vi "SRV_Comm.vi"(3 "TCP Settings":T1={"Method"=enum."General", "bytes to read"=2000, "timeout ms (1000)"=1000}, 4 "Command Sent":string, 5 "SRV In":refnum<k5>) -> (0 "Full comm":string, 1 "Reply":string, 2 "SRV Out":refnum<k5>)   [LabVIEW 2009]
uses:
  SRVGlobals.vi
  TCP_Communication/SRV_TCP Settings.ctl
  TCP_Communication/SRV_Package Methods.ctl
panel:
  # "This LabVIEW item is deprecated.\n\nIt is believed to be unused and will be removed in a future version of SRV."
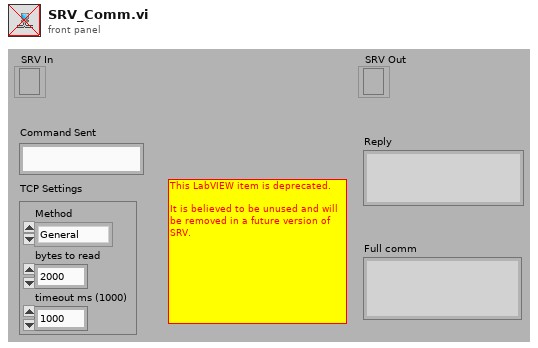
[diagram p1: front panel]
types:
  T1 = typedef "SRV_TCP Settings.ctl" = cluster{"Method":T2, "bytes to read":i32, "timeout ms (1000)":i32}
  T2 = typedef "SRV_Package Methods.ctl" = enum16{"General", "Standard", "CRLF", "Image", "HTML"}
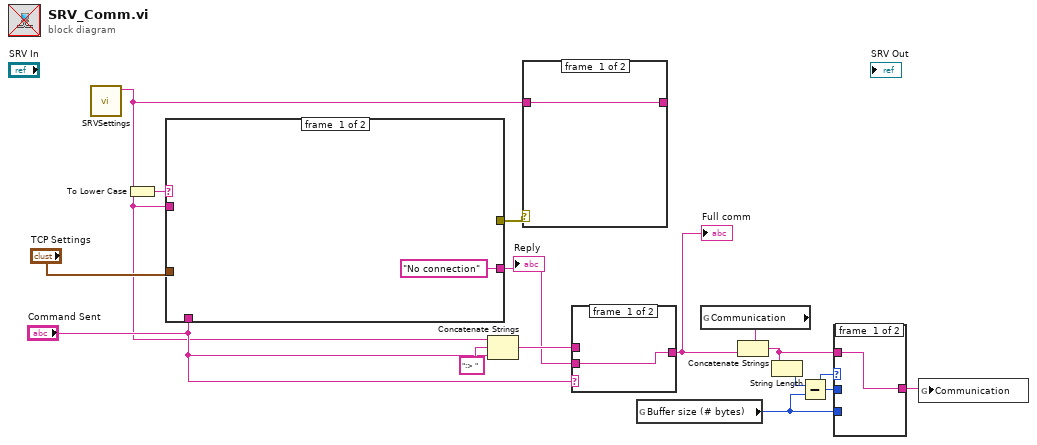
[diagram p0: block diagram]
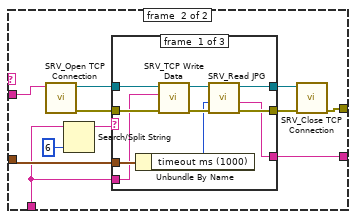
[diagram p2: hidden frame]
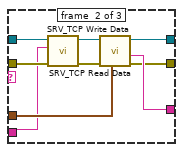
[diagram p3: hidden frame]
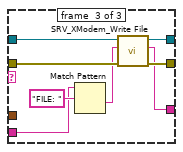
[diagram p4: hidden frame]
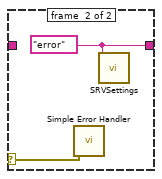
[diagram p5: hidden frame]
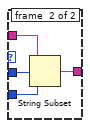
[diagram p6: hidden frame]
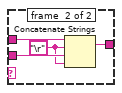
[diagram p7: hidden frame]
diagram:
  n1 = call "SRVSettings.vi"() -> ("SRV IP Address out"=w2:string, "SRV IP Address"=w5:string)  [unwired: 8 in, 2 out]
  n2 = To Lower Case(string=w2) -> (all lower case string=w1:string)
  n3 = case shown="Default" w1 {
    tunnel: "TCP Settings" -> [_ w25]
    tunnel: ["No connection" ("reply to upload") w24] -> w10
    tunnel: "Command Sent" -> [_ w22]
    tunnel: [_ w20] -> w4
    tunnel: w2 -> [_ w19]
    frame #0 {
    }
    frame #1 {
      n4 = call "SRV_Open TCP Connection.vi"("IP address"=w19) -> ("error out"=w26:errorcluster, "connection ID"=w27:refnum<k5>)  [unwired: 9 in]
      n5 = Search/Split String(string=w22, offset (0)=6) -> (substring before match=w23:string)  [unwired: 1 in, 2 out]
      n6 = case shown="Default" w23 {
        tunnel: w26 -> [w34 w44 w54]
        tunnel: w27 -> [w36 w45 w56]
        tunnel: [w39 w48 w55] -> w29
        tunnel: [w37 w47 w52] -> w24
        tunnel: [w38 w46 w53] -> w28
        tunnel: w25 -> [w32 w41 _]
        tunnel: w22 -> [w30 w40 w49]
        frame #0 {
          n7 = Unbundle By Name(w32) -> ("timeout ms (1000)"=w31:i32)
          n8 = call "SRV_TCP Write Data.vi"("error in"=w34, "data in"=w30, "connection ID"=w36) -> ("error out"=w33:errorcluster, "connection ID out"=w35:refnum<k5>)  [unwired: 6 in, 1 out]
          n9 = call "SRV_Read JPG.vi"("error in"=w33, "timeout ms (25000)"=w31, "connection ID in"=w35) -> ("error out"=w38:errorcluster, "data out"=w37:string, "connection ID"=w39:refnum<k5>)  [unwired: 6 in]
        }
        frame #1 {
          n10 = call "SRV_TCP Write Data.vi"("error in"=w44, "data in"=w40, "connection ID"=w45) -> ("error out"=w42:errorcluster, "connection ID out"=w43:refnum<k5>)  [unwired: 6 in, 1 out]
          n11 = call "SRV_TCP Read Data.vi"("TCP Settings"=w41, "error in"=w42, "connection ID in"=w43) -> ("error out"=w46:errorcluster, "data out"=w47:string, "connection ID"=w48:refnum<k5>)  [unwired: 2 in, 1 out]
        }
        frame #2 {
          n12 = Match Pattern(string=w49, regular expression="FILE: " ("string")) -> (after substring=w50:string)  [unwired: 1 in, 3 out]
          n13 = call "SRV_XModem_Write File.vi"("error in"=w54, "file contents"=w50, "connection ID in"=w56) -> ("error out"=w53:errorcluster, "reply to upload"=w52:string, "connection ID"=w55:refnum<k5>)  [unwired: 4 in, 2 out]
        }
      }
      n14 = call "SRV_Close TCP Connection.vi"("error in"=w28, "connection ID"=w29) -> ("error out"=w20:errorcluster)  [unwired: 9 in]
    }
  }
  "Reply" <- w10
  n15 = Concatenate Strings(w2, ":> " ("string"), "Command Sent") -> (w13:string)
  n16 = case shown="Error" w4 {
    selector: w4 -> [_ w59]
    tunnel: w2 -> [w57 _]
    tunnel: [w57 w58] -> w3
    frame #0 {
    }
    frame #1 {
      w58 = "error" ("SRV Out")
      n17 = call <vilib>:"Simple Error Handler.vi"("error in (no error)"=w59) -> ()  [unwired: 4 in, 5 out]
      n18 = call "SRVSettings.vi"("SRV IP Address"=w58) -> ()  [unwired: 8 in, 3 out]
    }
  }
  n19 = case shown="Default" "Command Sent" {
    tunnel: [w60 w64] -> w7
    tunnel: w13 -> [_ w63]
    tunnel: w10 -> [w60 w62]
    frame #0 {
    }
    frame #1 {
      w61 = "\r"
      n20 = Concatenate Strings(w63, w61, w62, w61) -> (w64:string)
    }
  }
  "Full comm" <- w7
  n21 = global read "SRVGlobals.vi" "Buffer size (# bytes)"() -> (w15:i32)
  n22 = global read "SRVGlobals.vi" "Communication"() -> (w9:string)
  n23 = Concatenate Strings(w9, w7) -> (w8:string)
  n24 = String Length(string=w8) -> (length=w16:i32)
  n25 = Subtract(x=w16, y=w15) -> (x-y=w14:i32)
  n26 = case shown="0.." w14 {
    tunnel: [w65 w69] -> w17
    tunnel: w8 -> [w65 w68]
    tunnel: w15 -> [_ w67]
    tunnel: w14 -> [_ w66]
    frame #0 {
    }
    frame #1 {
      n27 = String Subset(string=w68, offset (0)=w66, length (rest)=w67) -> (substring=w69:string)
    }
  }
  n28 = global write "SRVGlobals.vi" "Communication"(w17) -> ()
